vi "SetCol.vi"(4 "ModeCol Index":i32=2, 5 "Col Array Ref in":refnum<vi>, 6 "Cell Position":T1, 7 "Table History ref":refnum<vi>, 8 "error in (no error)":errorcluster, 9 "Table CtlRef In":refnum<vi>, 10 "SetTo":string, 11 "Column in":refnum<class "Column.lvclass">) -> (0 "error out":errorcluster, 1 "Table CtlRef Out":refnum<vi>, 2 "Num Rows":i32, 3 "Column out":refnum<class "Column.lvclass">)   [LabVIEW 2013, in "Column.lvclass"]
uses:
  Column.lvclass
  <vilib>/Utility/miscctls.llb/LVRowAndColumnTypeDef.ctl
  TypeDefs/TableHistory.ctl
  TypeDefs/TableArray.ctl
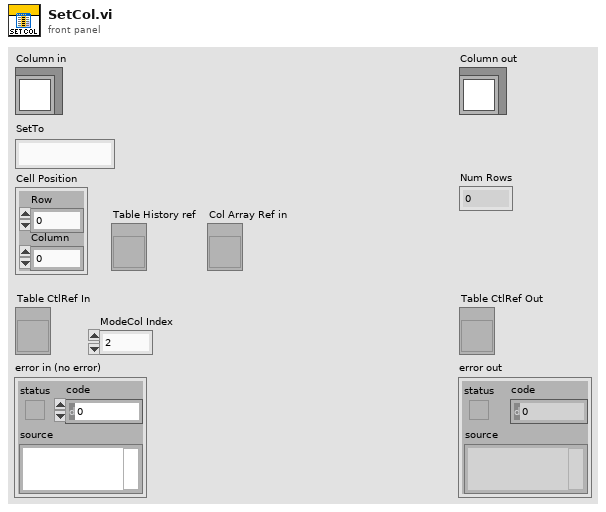
[diagram p1: front panel]
types:
  T1 = typedef "LVRowAndColumnTypeDef.ctl" = cluster{"Row":i32, "Column":i32}
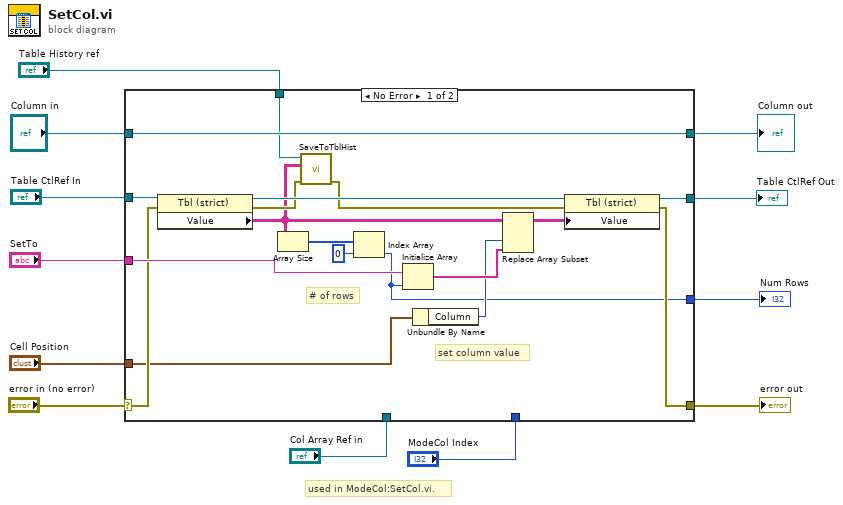
[diagram p0: block diagram]
diagram:
  # "used in ModeCol:SetCol.vi."
  n1 = case shown="No Error" "error in (no error)" {
    selector: "error in (no error)" -> [w26 w33]
    tunnel: [w28 w33] -> w11
    tunnel: [w18 w32] -> w5
    tunnel: "Column in" -> [w18 w32]
    tunnel: [w29 w31] -> w10
    tunnel: "Table CtlRef In" -> [w27 w31]
    tunnel: "SetTo" -> [w30 _]
    tunnel: "Cell Position" -> [w21 _]
    tunnel: [w17 _] -> w4
    tunnel: "Table History ref" -> [w13 _]
    tunnel: "Col Array Ref in" -> [_ _]
    tunnel: "ModeCol Index" -> [_ _]
    frame No Error {
      # "set column value"
      # "# of rows"
      n2 = property class="Tbl (strict)"(reference=w27, error in=w26) -> (reference out=w19:refnum<vi>, error out=w16:errorcluster, "Value"=w14:string[][])
      n3 = Array Size(array=w14) -> (size(s)=w24:i32[])
      n4 = call "SaveToTblHist.vi"("error in (no error)"=w16, "OldTable (reset)"=w14, "Table History ref"=w13) -> ("error out"=w15:errorcluster)  [unwired: 8 in]
      n5 = Index Array(array=w24, index=0) -> (element=w17:i32)
      n6 = Initialize Array "Initialize Array"(w30, w17) -> (w22:string[])
      n7 = Unbundle By Name(w21) -> ("Column"=w20:i32)
      n8 = Replace Array Subset(array=w14, new element=w22, index (col)=w20) -> (w25:string[][])  [unwired: 1 in]
      n9 = property class="Tbl (strict)"(reference=w19, error in=w15, "Value"=w25) -> (reference out=w29:refnum<vi>, error out=w28:errorcluster)
    }
    frame Error {
    }
  }
  "error out" <- w11
  "Table CtlRef Out" <- w10
  "Column out" <- w5
  "Num Rows" <- w4
